vi "SMB.vi"(1 "IP":string, 2 "In":variant, 3 "Mode":u32(ring) items=["Open", "Close", "Begin", "End", "Get", "Set"]) -> (0 "Out":variant)   [LabVIEW 2014]
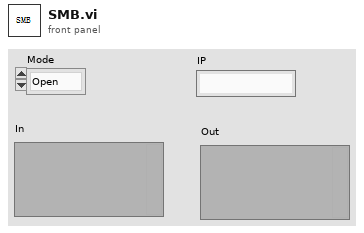
[diagram p1: front panel]
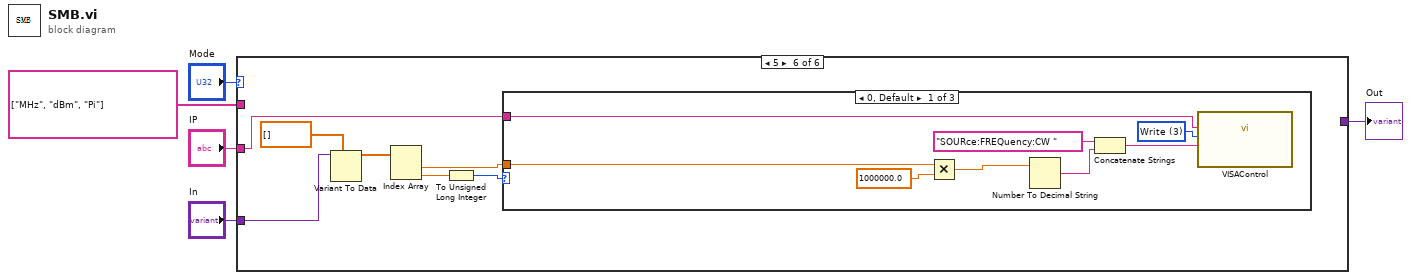
[diagram p0: block diagram]
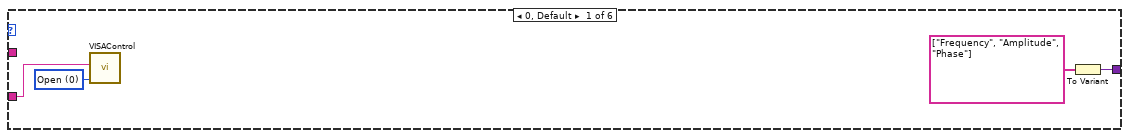
[diagram p2: hidden frame]
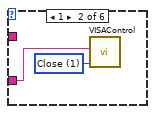
[diagram p3: hidden frame]
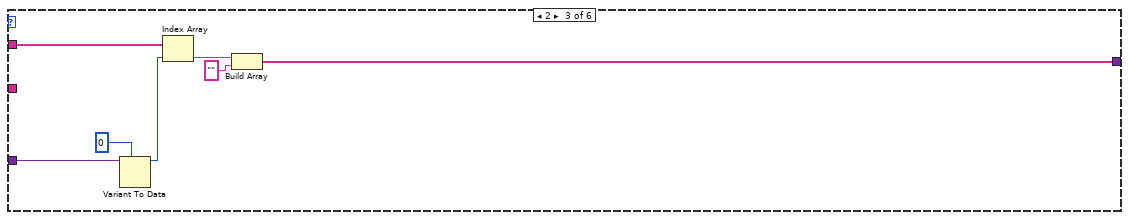
[diagram p4: hidden frame]
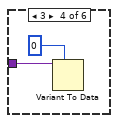
[diagram p5: hidden frame]
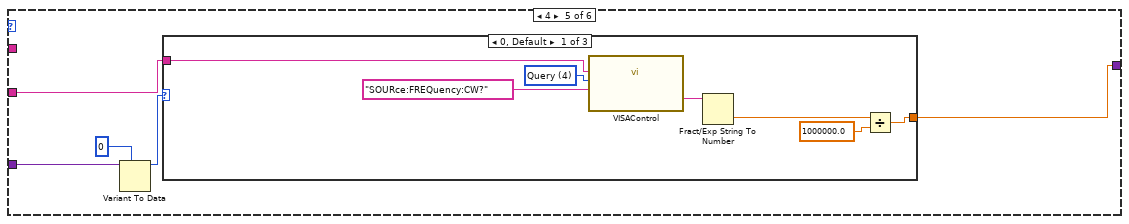
[diagram p6: hidden frame]
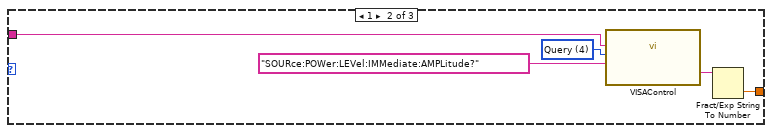
[diagram p7: hidden frame]
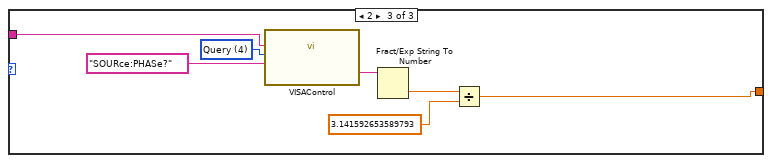
[diagram p8: hidden frame]
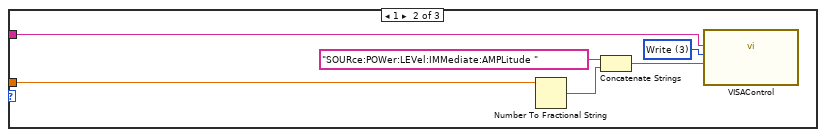
[diagram p9: hidden frame]
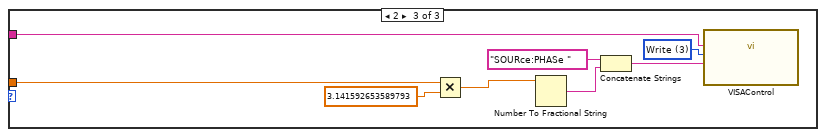
[diagram p10: hidden frame]
diagram:
  n1 = case shown="5" "Mode" {
    tunnel: "In" -> [_ _ w18 w19 w24 w50]
    tunnel: [w8 _ w12 _ w21 _] -> w3
    tunnel: "IP" -> [w7 w11 _ _ w22 w45]
    tunnel: string[] ["MHz", "dBm", "Pi"] ("Strings []") -> [_ _ w15 _ _ _]
    frame 0, Default {
      w6 = u32 0 items=["Open", "Close", "Read", "Write", "Query"] ("Mode")
      n2 = call "VISAControl.vi"("IP"=w7, "Mode"=w6) -> ()  [unwired: 3 in, 2 out]
      n3 = To Variant(anything=string[] ["Frequency", "Amplitude", "Phase"] ("Strings []")) -> (Variant=w8:variant)
    }
    frame 1 {
      w10 = u32 1 items=["Open", "Close", "Read", "Write", "Query"] ("Mode")
      n4 = call "VISAControl.vi"("IP"=w11, "Mode"=w10) -> ()  [unwired: 3 in, 2 out]
    }
    frame 2 {
      n5 = Variant To Data(type=0, Variant=w18) -> (data=w14:i32)  [unwired: 1 in, 1 out]
      n6 = Index Array(array=w15, index=w14) -> (element=w13:string)
      n7 = Build Array(w13, "") -> (w12:string[])
    }
    frame 3 {
      n8 = Variant To Data(type=0, Variant=w19) -> ()  [unwired: 1 in, 2 out]
    }
    frame 4 {
      n9 = Variant To Data(type=u32 0, Variant=w24) -> (data=w23:u32)  [unwired: 1 in, 1 out]
      n10 = case shown="0, Default" w23 {
        tunnel: w22 -> [w27 w34 w41]
        tunnel: [w26 w33 w38] -> w21
        frame 0, Default {
          w31 = u32 4 items=["Open", "Close", "Read", "Write", "Query"] ("Mode")
          n11 = call "VISAControl.vi"("IP"=w27, "Mode"=w31, "Write Buffer"="SOURce:FREQuency:CW?") -> ("Read Buffer"=w29:string)  [unwired: 2 in, 1 out]
          n12 = Fract/Exp String To Number(string=w29) -> (number=w28:dbl)  [unwired: 3 in, 1 out]
          n13 = Divide(x=w28, y=1000000.0) -> (x/y=w26:dbl)
        }
        frame 1 {
          w37 = u32 4 items=["Open", "Close", "Read", "Write", "Query"] ("Mode")
          n14 = call "VISAControl.vi"("IP"=w34, "Mode"=w37, "Write Buffer"="SOURce:POWer:LEVel:IMMediate:AMPLitude?") -> ("Read Buffer"=w35:string)  [unwired: 2 in, 1 out]
          n15 = Fract/Exp String To Number(string=w35) -> (number=w33:dbl)  [unwired: 3 in, 1 out]
        }
        frame 2 {
          w44 = u32 4 items=["Open", "Close", "Read", "Write", "Query"] ("Mode")
          n16 = call "VISAControl.vi"("IP"=w41, "Mode"=w44, "Write Buffer"="SOURce:PHASe?") -> ("Read Buffer"=w42:string)  [unwired: 2 in, 1 out]
          n17 = Fract/Exp String To Number(string=w42) -> (number=w39:dbl)  [unwired: 3 in, 1 out]
          n18 = Divide(x=w39, y=3.141592653589793) -> (x/y=w38:dbl)
        }
      }
    }
    frame 5 {
      n19 = Variant To Data(type=dbl[] [] ("appended array"), Variant=w50) -> (data=w49:dbl[])  [unwired: 1 in, 1 out]
      n20 = Index Array(array=w49) -> (element #1=w46:dbl, element #2=w48:dbl)  [unwired: 2 in]
      n21 = To Unsigned Long Integer(number=w48) -> (unsigned 32bit integer=w47:u32)
      n22 = case shown="0, Default" w47 {
        tunnel: w46 -> [w59 w62 w72]
        tunnel: w45 -> [w52 w60 w66]
        frame 0, Default {
          w57 = u32 3 items=["Open", "Close", "Read", "Write", "Query"] ("Mode")
          n23 = Multiply(x=w59, y=1000000.0) -> (x*y=w53:dbl)
          n24 = Number To Decimal String(number=w53) -> (decimal integer string=w55:string)  [unwired: 1 in]
          n25 = Concatenate Strings("SOURce:FREQuency:CW " ("Write Buffer"), w55) -> (w54:string)
          n26 = call "VISAControl.vi"("IP"=w52, "Mode"=w57, "Write Buffer"=w54) -> ()  [unwired: 2 in, 2 out]
        }
        frame 1 {
          w65 = u32 3 items=["Open", "Close", "Read", "Write", "Query"] ("Mode")
          n27 = Number To Fractional String(number=w62) -> (F-format string=w61:string)  [unwired: 3 in]
          n28 = Concatenate Strings("SOURce:POWer:LEVel:IMMediate:AMPLitude " ("Write Buffer"), w61) -> (w63:string)
          n29 = call "VISAControl.vi"("IP"=w60, "Mode"=w65, "Write Buffer"=w63) -> ()  [unwired: 2 in, 2 out]
        }
        frame 2 {
          w70 = u32 3 items=["Open", "Close", "Read", "Write", "Query"] ("Mode")
          n30 = Multiply(x=w72, y=3.141592653589793) -> (x*y=w71:dbl)
          n31 = Number To Fractional String(number=w71) -> (F-format string=w67:string)  [unwired: 3 in]
          n32 = Concatenate Strings("SOURce:PHASe " ("Write Buffer"), w67) -> (w68:string)
          n33 = call "VISAControl.vi"("IP"=w66, "Mode"=w70, "Write Buffer"=w68) -> ()  [unwired: 2 in, 2 out]
        }
      }
    }
  }
  "Out" <- w3
